vi "Read Output.vi"(8 "error in (no error)":errorcluster, 10 "Channel (1: Channel 1)":i32(ring)=1 items=["Channel 1"=1, "Channel 2"=2, "Channel 3"=3], 11 "VISA resource name":refnum<visa-resource-name>) -> (0 "error out":errorcluster, 1 "Actual Current Level (A)":dbl format="%.3g", 2 "Actual Voltage Level (V)":dbl format="%.3g", 3 "VISA resource name out":refnum<visa-resource-name>)   [LabVIEW 2009, in "Agilent E363X Series.lvlib"]
doc: "Returns the Actual Voltage Level and Actual Current Level for a desired channel."
uses:
  <instrlib>/Agilent E363X Series/Agilent E363X Series.lvlib
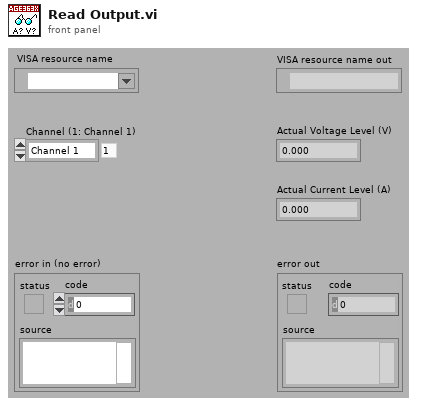
[diagram p1: front panel]
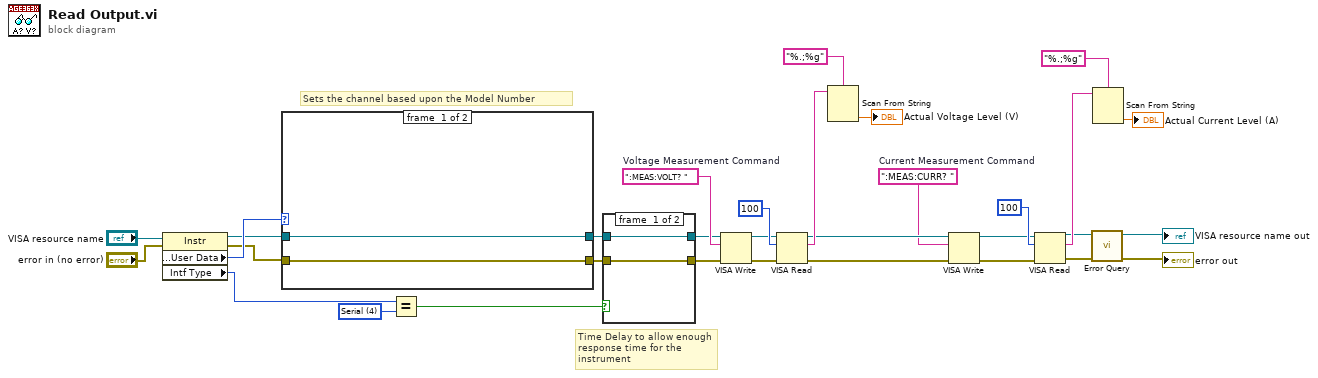
[diagram p0: block diagram]
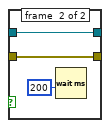
[diagram p2: hidden frame]
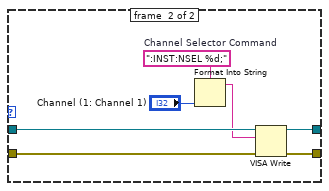
[diagram p3: hidden frame]
diagram:
  w7 = u16 4 items=["GPIB"=1, "VXI"=2, "GPIB-VXI"=3, "Serial"=4, "PXI"=5, "TCPIP"=6, "USB"=7] ("Interface Information:Interface Type")
  w22 = ":MEAS:CURR? "  # Current Measurement Command
  w21 = ":MEAS:VOLT? "  # Voltage Measurement Command
  # "Time Delay to allow enough response time for the instrument"
  # "Sets the channel based upon the Model Number"
  n1 = property on="Property Node" class="Instr"(reference="VISA resource name", error in="error in (no error)") -> (reference out=w17:refnum<visa-resource-name>, error out=w16:errorcluster, "General Settings:User Data"=w18:u32, "Intf Type"=w6:u16)
  n2 = case shown="3631, Default" w18 {
    tunnel: [w34 w39] -> w4
    tunnel: [w33 w38] -> w2
    tunnel: w17 -> [w34 w37]
    tunnel: w16 -> [w33 w36]
    frame #0 {
    }
    frame #1 {
      w40 = ":INST:NSEL %d;"  # Channel Selector Command
      n3 = Format Into String(format string=w40, "Channel (1: Channel 1)") -> (resulting string=w35:string)  [unwired: 2 in, 1 out]
      n4 = VISA Write(VISA resource name=w37, write buffer=w35, error in (no error)=w36) -> (VISA resource name out=w39:refnum<visa-resource-name>, error out=w38:errorcluster)  [unwired: 1 out]
    }
  }
  n5 = Equal?(x=w6, y=w7) -> (x = y?=w5:bool)
  n6 = case shown="True" w5 {
    tunnel: [w43 w45] -> w3
    tunnel: w4 -> [w43 w45]
    tunnel: [w42 w44] -> w1
    tunnel: w2 -> [w42 w44]
    frame #0 {
    }
    frame #1 {
      n7 = Wait (ms)(milliseconds to wait=u32 200) -> ()  [unwired: 1 out]
    }
  }
  n8 = VISA Write(VISA resource name=w3, write buffer=w21, error in (no error)=w1) -> (VISA resource name out=w15:refnum<visa-resource-name>, error out=w14:errorcluster)  [unwired: 1 out]
  n9 = VISA Read(VISA resource name=w15, byte count=u32 100, error in (no error)=w14) -> (VISA resource name out=w23:refnum<visa-resource-name>, read buffer=w30:string, error out=w24:errorcluster)  [unwired: 1 out]
  n10 = Scan From String(format string="%.;%g", input string=w30) -> (output 1=→"Actual Voltage Level (V)":dbl)  [unwired: 3 in, 3 out]
  n11 = VISA Write(VISA resource name=w23, write buffer=w22, error in (no error)=w24) -> (VISA resource name out=w13:refnum<visa-resource-name>, error out=w12:errorcluster)  [unwired: 1 out]
  n12 = VISA Read(VISA resource name=w13, byte count=u32 100, error in (no error)=w12) -> (VISA resource name out=w9:refnum<visa-resource-name>, read buffer=w27:string, error out=w8:errorcluster)  [unwired: 1 out]
  n13 = call <instrlib>:"Error Query.vi"("error in (no error)"=w8, "VISA resource name"=w9) -> ("error out"=→"error out":errorcluster, "VISA resource name out"=→"VISA resource name out":refnum<visa-resource-name>)  [unwired: 6 in, 2 out]
  n14 = Scan From String(format string="%.;%g", input string=w27) -> (output 1=→"Actual Current Level (A)":dbl)  [unwired: 3 in, 3 out]
